vi "Receive Command.vi"(8 "error in (no error)":errorcluster, 9 "timeout in ms (0)":i32 format="%d ms", 11 "Transceiver Thread in":refnum<class "Transceiver Thread.lvclass">) -> (0 "error out":errorcluster, 1 "timed out?":bool, 2 "command":T1={"Command"=enum."Receive", "Command Parameters"={"arg1"=0, "arg2"=0}}, 3 "Transceiver Thread out":refnum<class "Transceiver Thread.lvclass">)   [LabVIEW 2017, in "Data Sharing Framework Engine.lvlib" / "Transceiver Thread.lvclass"]
uses:
  Transceiver Thread.lvclass
  Interfaces/Transceiver Interface/Command Data.ctl
  Interfaces/Transceiver Interface/Command.ctl
  Interfaces/Transceiver Interface/Command Parameters.ctl
  Transceiver Thread.lvclass/Transceiver Thread.ctl
  Interfaces/Engine Interface/Engine Interface.lvclass/Engine Interface.ctl
  Debug/Debug Flags FIFO/Debug Flags FIFO.lvclass/Debug Flags FIFO.ctl
  Interfaces/Transceiver Interface/Read Transceiver Command.vi
  Interfaces/Engine Interface/Read Command.vi
  Interfaces/Engine Interface/Get Command FIFO.vi
  Interfaces/Engine Interface/Get Debug Flags.vi
  Interfaces/Engine Interface/Read 16B RT FIFO.vi
  Debug/Debug Flags FIFO/Get Infinite Timeouts.vi
  Interfaces/Transceiver Interface/Transceiver Interface.lvclass
  C:/github/data-sharing-framework/Source/Data Sharing Framework Core/Engine/Interfaces/Engine Interface/Engine Interface.lvclass
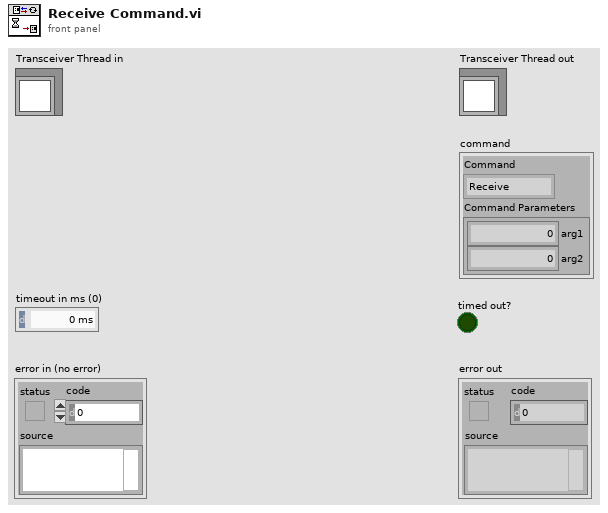
[diagram p1: front panel]
types:
  T1 = typedef "Data Sharing Framework Engine.lvlib/Transceiver Interface.lvclass/Command Data.ctl" = cluster{"Command":T2, "Command Parameters":T3}
  T2 = typedef "Data Sharing Framework Engine.lvlib/Transceiver Interface.lvclass/Command.ctl" = enum8{"Set Base Pointer", "Receive", "Transmit", "Shutdown"}
  T3 = typedef "Data Sharing Framework Engine.lvlib/Transceiver Interface.lvclass/Command Parameters.ctl" = cluster{"arg1":u64, "arg2":u64}
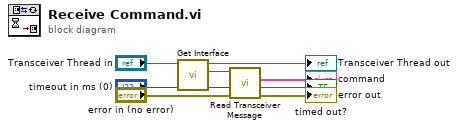
[diagram p0: block diagram]
diagram:
  n1 = call "Get Interface.vi"("Transceiver Thread in"="Transceiver Thread in") -> ("Interface"=w7:refnum<class "Transceiver Interface.lvclass">, "Transceiver Thread out"=→"Transceiver Thread out":refnum<class "Transceiver Thread.lvclass">)  [unwired: 9 in]
  n2 = call-poly "Read Transceiver Message.vi"("error in (no error)"="error in (no error)", "timeout in ms (0)"="timeout in ms (0)", "Transceiver Interface in"=w7) -> ("error out"=→"error out":errorcluster, "empty?"=→"timed out?":bool, "command"=→"command":T1)  [unwired: 4 in, 2 out]
